vi "Write Export's Build Spec Name.vi"(8 "error in (no error)":errorcluster, 10 "Export's Build Spec Name":string, 11 "NI Build Specification_LV in":refnum<class "NI Build Specification_LV.lvclass">) -> (0 "error out":errorcluster, 3 "NI Build Specification_LV out":refnum<class "NI Build Specification_LV.lvclass">)   [LabVIEW 2017, in "CL_G3_VIComponentBuilder.lvlib" / "NI Build Specification_LV.lvclass"]
uses:
  NI Build Specification_LV.lvclass
  C:/Tool Chain Support/Software Module Builder/Source/Exports/Exports/Export.lvclass
  NI Build Specification_LV.lvclass/NI Build Specification_LV.ctl
  Exports/Export.lvclass/Export.ctl
  Exports/Export.lvclass
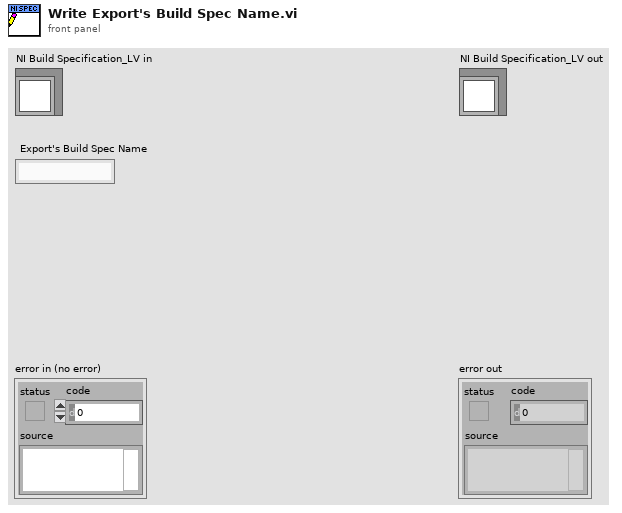
[diagram p1: front panel]
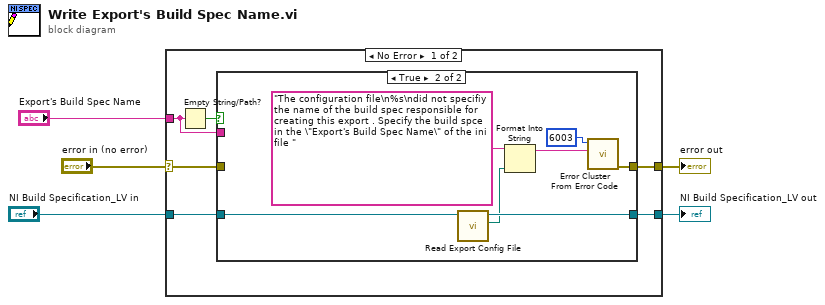
[diagram p0: block diagram]
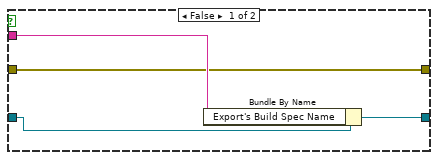
[diagram p2: hidden frame]
diagram:
  n1 = case shown="No Error" "error in (no error)" {
    selector: "error in (no error)" -> [w6 w23]
    tunnel: [w7 w23] -> w4
    tunnel: [w10 w24] -> w2
    tunnel: "NI Build Specification_LV in" -> [w11 w24]
    tunnel: "Export's Build Spec Name" -> [w9 _]
    frame No Error {
      n2 = Empty String/Path?(string/path=w9) -> (empty?=w8:bool)
      n3 = case shown="True" w8 {
        tunnel: w11 -> [w15 w18]
        tunnel: [w14 w17] -> w10
        tunnel: w9 -> [w13 _]
        tunnel: [w12 w22] -> w7
        tunnel: w6 -> [w12 _]
        frame False {
          n4 = Bundle By Name(cluster=w15, "Export's Build Spec Name"=w13) -> (w14:refnum<class "NI Build Specification_LV.lvclass">)
        }
        frame True {
          n5 = call "Read Export Config File.vi"("Export in"=w18) -> ("Export Definition File Path"=w16:path, "Export out"=w17:refnum<class "NI Build Specification_LV.lvclass">)  [unwired: 8 in, 1 out]
          n6 = Format Into String(format string="The configuration file\n%s\ndid not specifiy the name of the build spec responsible for creating this export . Specify the build spce in the \"Export's Build Spec Name\" of the ini file ", w16) -> (resulting string=w20:string)  [unwired: 2 in, 1 out]
          n7 = call <vilib>:"Error Cluster From Error Code.vi"("error message (\"\")"=w20, "error code (0)"=6003) -> ("error out"=w22:errorcluster)  [unwired: 7 in]
        }
      }
    }
    frame Error {
    }
  }
  "error out" <- w4
  "NI Build Specification_LV out" <- w2
